vi "PhotodiodeTester.vi"() -> ()   [LabVIEW 2015]
uses:
  <vilib>/LabVIEW Interface for Arduino/Type Defs/Board Type.ctl
  <vilib>/LabVIEW Interface for Arduino/Type Defs/Connection Type.ctl
  <vilib>/LabVIEW Interface for Arduino/LabVIEW Interface for Arduino.lvlib
panel:
  out "PWM Val":i32
  out "XY Graph":cluster{"Y":dbl[], "Y":dbl[]}[](graph)
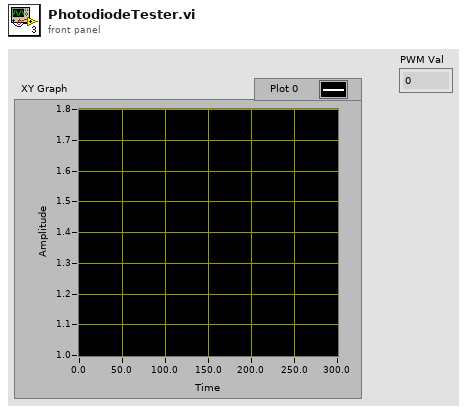
[diagram p1: front panel]
types:
  T1 = typedef "LabVIEW Interface for Arduino.lvlib/Connection Type.ctl" = enum8{"USB / Serial", "XBEE", "BlueSmirf (Bluetooth)"}
  T2 = typedef "LabVIEW Interface for Arduino.lvlib/Board Type.ctl" = enum16{"Uno", "Dimuelanove w/Atmega 328", "Mega 2560"}
  T3 = typedef "LabVIEW Interface for Arduino.lvlib/Arduino Resource.ctl" = cluster{"VISA resource":refnum<visa-resource-name>, "Board Type":T2, "Connection Type":enum8{"USB / Serial"}, "Bytes Per Packet (15)":u8}
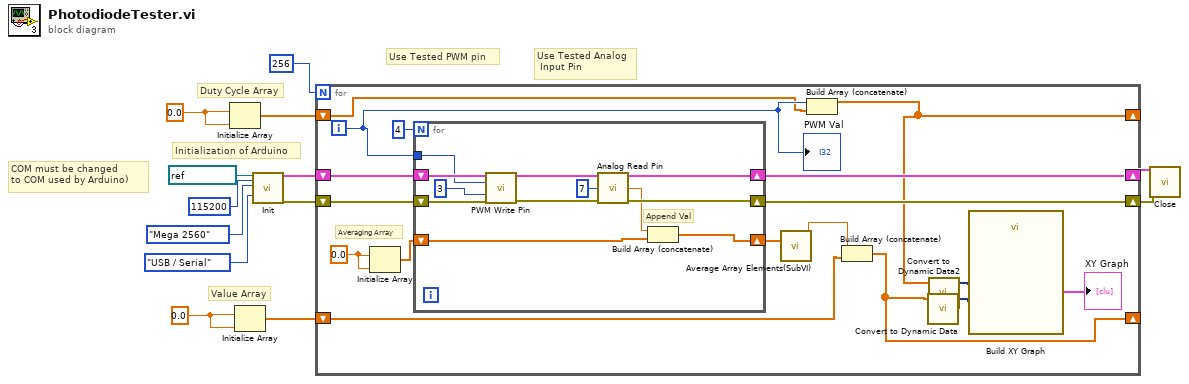
[diagram p0: block diagram]
diagram:
  w4 = 0.0 ("element")
  w6 = 0.0 ("element")
  # "Duty Cycle Array"
  # "Value Array"
  # "Use Tested Analog\n Input Pin"
  # "Use Tested PWM pin"
  # "COM must be changed \nto COM used by Arduino)"
  # "Initialization of Arduino"
  n1 = Initialize Array(w4, w4) -> (w3:dbl[])
  n2 = Initialize Array(w6, w6) -> (w5:dbl[])
  n3 = call <vilib>:"Init.vi"("VISA resource"=refnum<visa-resource-name> "COM10", "Baud Rate (115200)"=u32 115200, "Board Type (Uno)"=Board_Type."Mega 2560", "Connection Type (USB/Serial)"=Connection_Type."USB / Serial") -> ("Arduino Resource"=w8:T3, "error out"=w7:errorcluster)  [unwired: 14 in]
  n4 = for {
    N: 256 -> [_]
    shift-right: [w16] -> _
    shift-left: w5 -> [w23]
    shift-right: [w22] -> w2
    shift-left: w8 -> [w27]
    shift-right: [w21] -> w1
    shift-left: w7 -> [w26]
    shift-right: [w18] -> _
    shift-left: w3 -> [w14]
    i -> [w15]
    w29 = 0.0 ("element")
    # "Averaging Array"
    n5 = Initialize Array(w29, w29) -> (w28:dbl[])
    n6 = for {
      N: 4 -> [_]
      shift-right: [w31] -> w25
      shift-left: w28 -> [w33]
      shift-right: [w36] -> w22
      shift-left: w27 -> [w41]
      shift-right: [w35] -> w21
      shift-left: w26 -> [w42]
      tunnel: w15 -> [w40]
      # "Append Val"
      n7 = call <vilib>:"PWM Write Pin.vi"("Arduino Resource"=w41, "Duty Cycle (0 - 255)"=w40, "PWM Pin (3)"=u8 3, "error in"=w42) -> ("Arduino Resource"=w38:T3, "error out"=w37:errorcluster)  [unwired: 10 in]
      n8 = call <vilib>:"Analog Read Pin.vi"("Arduino Resource"=w38, "Analog Input Pin (0)"=u8 7, "error in"=w37) -> ("Arduino Resource"=w36:T3, "Voltage"=w32:dbl, "error out"=w35:errorcluster)  [unwired: 10 in]
      n9 = Build Array (concatenate)(w32, w33) -> (w31:dbl[])
    }
    n10 = call "Average Array Elements(SubVI).vi"("Array"=w25) -> ("Numeric"=w24:dbl)  [unwired: 10 in]
    n11 = Build Array (concatenate)(w15, w14) -> (w18:dbl[])
    n12 = Build Array (concatenate)(w24, w23) -> (w16:dbl[])
    n13 = call "Convert to Dynamic Data"("Array"=w16) -> ("Dynamic Data Type"=w19:dynamicdata)  [unwired: 3 in]
    n14 = call "Convert to Dynamic Data2"("Array"=w18) -> ("Dynamic Data Type"=w17:dynamicdata)  [unwired: 3 in]
    n15 = call "Build XY Graph"("Y Input"=w19, "X Input"=w17) -> ("XY Graph"=→"XY Graph":cluster{"X":dbl[], "Y":dbl[]}[])  [unwired: 8 in, 1 out]
    "PWM Val" <- w15
  }
  n16 = call <vilib>:"Close.vi"("Arduino Resource"=w2, "error in"=w1) -> ()  [unwired: 13 in, 1 out]
